vi "Get Actor Core.vi"(8 "error in (no error)":errorcluster, 11 "[V] Sys Cfg Base in":refnum<class "[V] Sys Cfg Base.lvclass">) -> (0 "error out":errorcluster, 3 "[V] Sys Cfg Base out":refnum<class "[V] Sys Cfg Base.lvclass">)   [LabVIEW 2023, in "[V] Sys Cfg Base.lvlib" / "[V] Sys Cfg Base.lvclass"]
uses:
  [V] Sys Cfg Base.lvclass
  [V] Sys Cfg Base.lvclass/[V] Sys Cfg Base.ctl
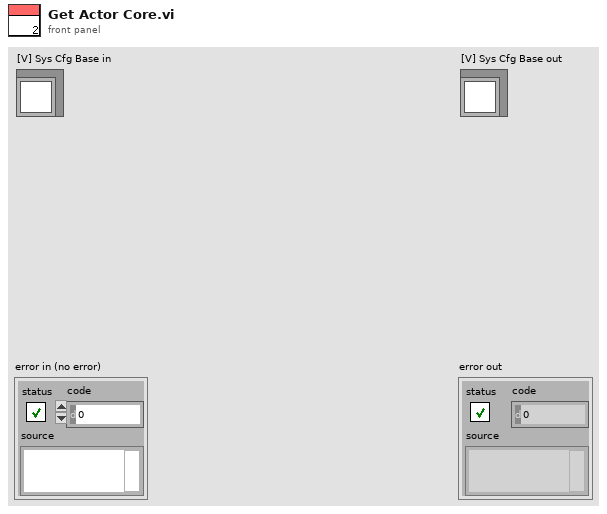
[diagram p1: front panel]
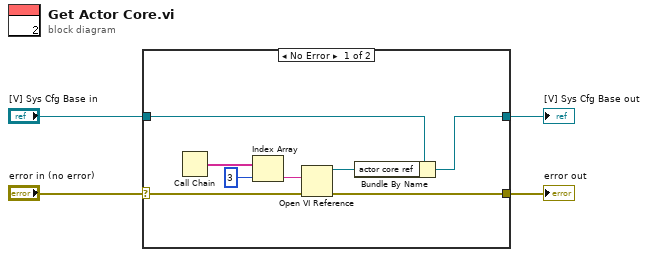
[diagram p0: block diagram]
diagram:
  n1 = case shown="No Error" "error in (no error)" {
    selector: "error in (no error)" -> [w9 w14]
    tunnel: [w8 w14] -> w3
    tunnel: [w5 w13] -> w1
    tunnel: "[V] Sys Cfg Base in" -> [w7 w13]
    frame No Error {
      n2 = Call Chain() -> (call chain=w12:string[])
      n3 = Index Array(array=w12, index=3) -> (element=w10:string)
      n4 = Open VI Reference(vi path=w10, error in (no error)=w9) -> (vi reference=w6:refnum<vi>, error out=w8:errorcluster)  [unwired: 4 in]
      n5 = Bundle By Name(cluster=w7, "actor core ref"=w6) -> (w5:refnum<class "[V] Sys Cfg Base.lvclass">)
    }
    frame Error {
    }
  }
  "error out" <- w3
  "[V] Sys Cfg Base out" <- w1
